vi "FABR-Init Data Files.vi"(0 "Runtime in":T1, 5 "Path":path, 7 "Frequency (kHz)":dbl[](array[numeric]), 9 "Level":dbl[](array[numeric]), 11 "error in (no error)":errorcluster, 12 "Save raw":bool, 13 "Fs (Hz)":dbl) -> (4 "Runtime out":T1, 15 "error out":errorcluster)   [LabVIEW 2020]
uses:
  Typedefs/FABR-Runtime Data.ctl
  Typedefs/FABR-Stimulus Ticket.ctl
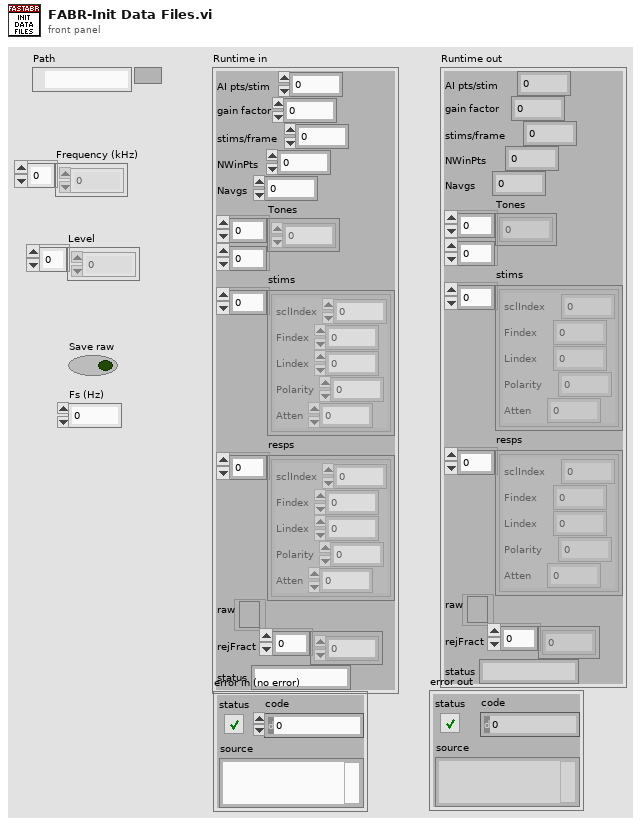
[diagram p1: front panel]
types:
  T1 = typedef "FABR-Runtime Data.ctl" = cluster{"AI pts/stim":i32, "gain factor":dbl, "stims/frame":i32, "NWinPts":i32, "Navgs":i32, "Tones":dbl[][], "stims":T2[], "resps":T2[], "raw":refnum<file>, "rejFract":dbl[], "status":string}
  T2 = typedef "FABR-Stimulus Ticket.ctl" = cluster{"sclIndex":i32, "Findex":i32, "Lindex":i32, "Polarity":i32, "Atten":dbl}
  T3 = enum16{"open", "replace", "create", "open or create", "replace or create", "replace or create with confirmation"}
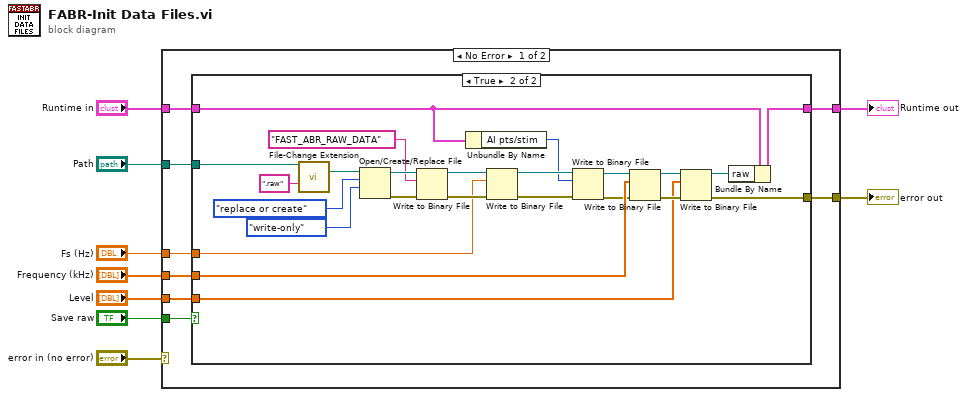
[diagram p0: block diagram]
diagram:
  n1 = case shown="No Error" "error in (no error)" {
    selector: "error in (no error)" -> [_ w44]
    tunnel: "Frequency (kHz)" -> [w14 _]
    tunnel: "Level" -> [w13 _]
    tunnel: "Runtime in" -> [w17 w43]
    tunnel: [w15 w43] -> w7
    tunnel: "Path" -> [w16 _]
    tunnel: "Save raw" -> [w11 _]
    tunnel: [w12 w44] -> w2
    tunnel: "Fs (Hz)" -> [w10 _]
    frame No Error {
      n2 = case shown="True" w11 {
        tunnel: w17 -> [w18 w21]
        tunnel: w16 -> [_ w42]
        tunnel: [w18 w35] -> w15
        tunnel: w14 -> [_ w33]
        tunnel: w13 -> [_ w30]
        tunnel: [_ w28] -> w12
        tunnel: w10 -> [_ w19]
        frame False {
        }
        frame True {
          n3 = call "File-Change Extension.vi"("Path"=w42, "new extension"=".raw") -> ("new path"=w40:path)  [unwired: 12 in, 1 out]
          n4 = Open/Create/Replace File(file path (use dialog)=w40, operation (0:open)=T3."replace or create", access (0:read/write)=enum16{"read/write", "read-only", "write-only"}."write-only") -> (refnum out=w37:refnum<file>, error out=w36:errorcluster)  [unwired: 3 in, 1 out]
          n5 = Write to Binary File(file (use dialog)=w37, data="FAST_ABR_RAW_DATA", error in=w36) -> (refnum out=w27:refnum<file>, error out=w26:errorcluster)  [unwired: 3 in, 1 out]
          n6 = Unbundle By Name(w21) -> ("AI pts/stim"=w20:i32)
          n7 = Write to Binary File(file (use dialog)=w27, data=w19, error in=w26) -> (refnum out=w25:refnum<file>, error out=w22:errorcluster)  [unwired: 3 in, 1 out]
          n8 = Write to Binary File(file (use dialog)=w25, data=w20, error in=w22) -> (refnum out=w24:refnum<file>, error out=w23:errorcluster)  [unwired: 3 in, 1 out]
          n9 = Write to Binary File(file (use dialog)=w24, data=w33, error in=w23) -> (refnum out=w32:refnum<file>, error out=w31:errorcluster)  [unwired: 3 in, 1 out]
          n10 = Write to Binary File(file (use dialog)=w32, data=w30, error in=w31) -> (refnum out=w29:refnum<file>, error out=w28:errorcluster)  [unwired: 3 in, 1 out]
          n11 = Bundle By Name(cluster=w21, "raw"=w29) -> (w35:T1)
        }
      }
    }
    frame Error {
    }
  }
  "Runtime out" <- w7
  "error out" <- w2
